vi "pl1000Ready.vi"(8 "error in (no error)":errorcluster, 11 "pl1000 handle":i16) -> (0 "error out":errorcluster, 2 "ready":bool, 3 "pl1000 handle out":i16)   [LabVIEW 2010]
doc: "This function indicates when pl1000Run has captured the requested number of samples."
uses:
  pl1000.dll
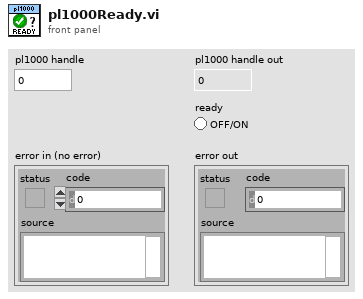
[diagram p1: front panel]
types:
  T1 = cluster{"status":bool, "code":u32, "source":string}
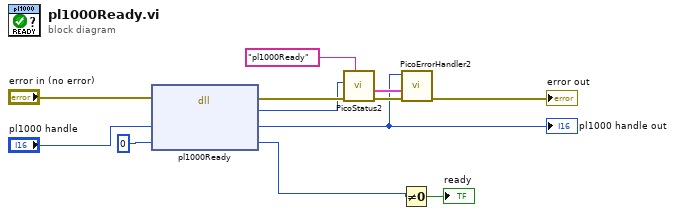
[diagram p0: block diagram]
diagram:
  n1 = dll-call lib="pl1000.dll" fn="pl1000Ready"(error in="error in (no error)", "handle"="pl1000 handle", "ready"=i16 0 ("maxValue")) -> (error out=w4:errorcluster, "status"=w3:u32, "handle"=w1:i16, "ready"=w9:i16)  [unwired: 2 in, 1 out]
  "pl1000 handle out" <- w1
  n2 = call "PicoStatus2.vi"("PICO source"="pl1000Ready", "Error in"=w4, "PICO STATUS"=w3) -> ("error out"=w7:errorcluster, "PICO_STATUS out"=w6:T1)  [unwired: 5 in]
  n3 = Not Equal To 0?(x=w9) -> (x != 0?=→"ready":bool)
  n4 = call "PicoErrorHandler2.vi"("error in (no error)"=w7, "PICO_STATUS in"=w6, "handle In"=w1) -> ("error out"=→"error out":errorcluster)  [unwired: 8 in]
